vi "_script_fix_vi broken in Tree__JKI_State_Machine_Helper.vi"   [LabVIEW 2014]
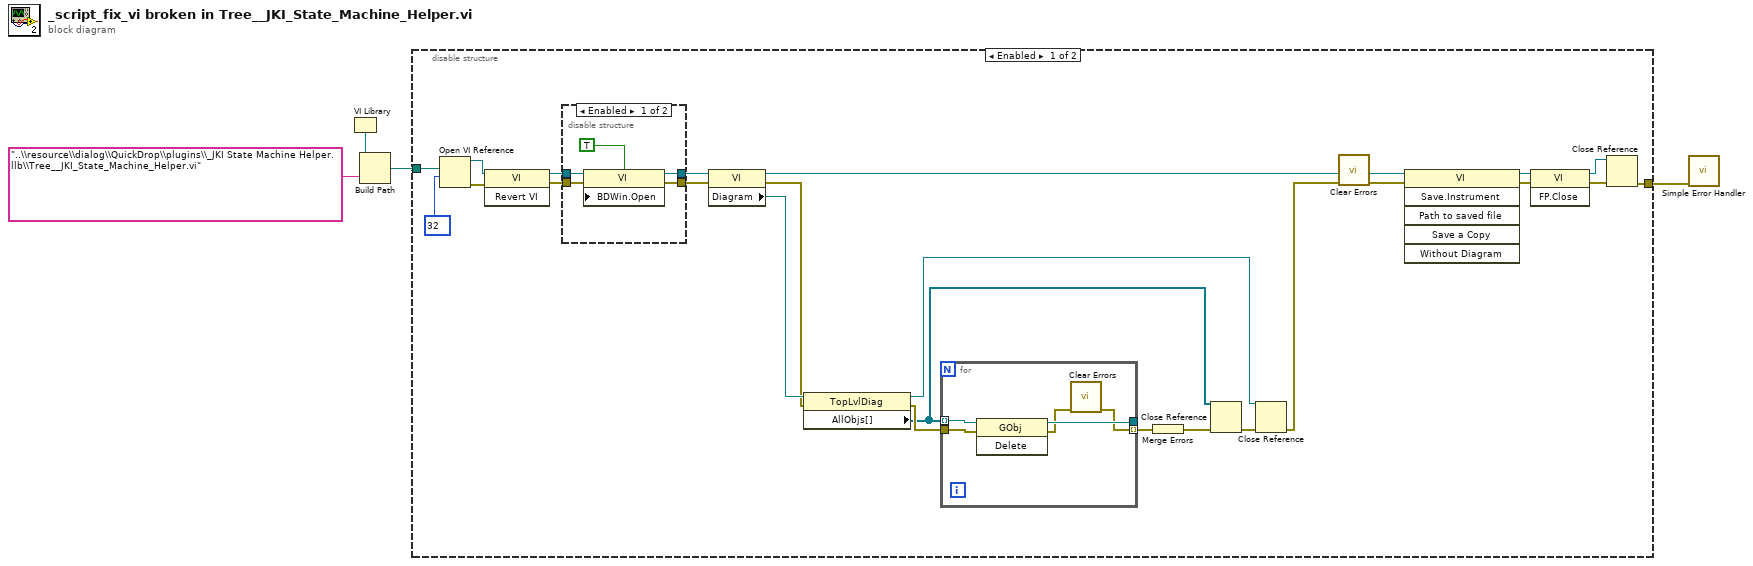
[diagram p0: block diagram]
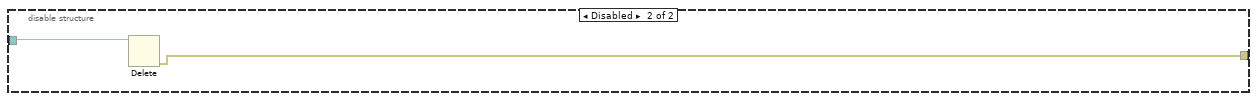
[diagram p3: hidden frame]
diagram:
  n1 = VI Library() -> (path=w4:path)
  n2 = Build Path(base path=w4, name or relative path="..\\resource\\dialog\\QuickDrop\\plugins\\_JKI State Machine Helper.llb\\Tree__JKI_State_Machine_Helper.vi") -> (appended path=w2:path)
  n3 = disable-structure shown="Enabled" {
    disable-tunnel: w2 -> [w26 w42]
    disable-tunnel: [w24 w41] -> w1
    frame Enabled {
      n4 = Open VI Reference(vi path=w26, options=32) -> (vi reference=w27:refnum<vi>, error out=w28:errorcluster)  [unwired: 4 in]
      n5 = invoke class="VI" method="Revert VI"(reference=w27, error in=w28) -> (reference out=w16:refnum<vi>, error out=w15:errorcluster)  [unwired: 1 in, 1 out]
      n6 = disable-structure shown="Enabled" {
        disable-tunnel: w16 -> [w33 w35]
        disable-tunnel: w15 -> [w32 w34]
        disable-tunnel: [w31 w35] -> w14
        disable-tunnel: [w30 w34] -> w13
        frame Enabled {
          n7 = property class="VI"(reference=w33, error in=w32, "BDWin.Open"=TRUE ("Block Diagram Window:Open")) -> (reference out=w31:refnum<vi>, error out=w30:errorcluster)
        }
        frame Disabled {
        }
      }
      n8 = property class="VI"(reference=w14, error in=w13) -> (reference out=w25:refnum<vi>, error out=w22:errorcluster, "Diagram"=w23:refnum<vi>)
      n9 = property class="TopLvlDiag"(reference=w23, error in=w22) -> (reference out=w18:refnum<vi>, error out=w21:errorcluster, "AllObjs[]"=w20:refnum<vi>[])
      n10 = for {
        tunnel: w20 -> [w40] mode=indexing
        tunnel: w21 -> [w39]
        tunnel: [w38] -> _
        tunnel: [w36] -> w7 mode=indexing
        n11 = invoke class="GObj" method="Delete"(reference=w40, error in=w39) -> (reference out=w38:refnum<vi>, error out=w37:errorcluster)  [unwired: 1 in, 1 out]
        n12 = call <vilib>:"Clear Errors.vi"("error in (no error)"=w37) -> ("error out"=w36:errorcluster)  [unwired: 5 in, 1 out]
      }
      n13 = Merge Errors(w7) -> (w6:errorcluster)
      n14 = Close Reference(reference=w20, error in (no error)=w6) -> (error out=w19:errorcluster)
      n15 = Close Reference(reference=w18, error in (no error)=w19) -> (error out=w17:errorcluster)
      n16 = call <vilib>:"Clear Errors.vi"("error in (no error)"=w17) -> ("error out"=w8:errorcluster)  [unwired: 5 in, 1 out]
      n17 = invoke class="VI" method="Save.Instrument"(reference=w25, error in=w8) -> (reference out=w10:refnum<vi>, error out=w12:errorcluster)  [unwired: 4 in, 4 out]
      n18 = invoke class="VI" method="FP.Close"(reference=w10, error in=w12) -> (reference out=w9:refnum<vi>, error out=w11:errorcluster)  [unwired: 1 in, 1 out]
      n19 = Close Reference(reference=w9, error in (no error)=w11) -> (error out=w24:errorcluster)
    }
    frame Disabled {
      n20 = Delete(path (use dialog)=w42) -> (error out=w41:errorcluster)  [unwired: 4 in, 2 out]
    }
  }
  n21 = call <vilib>:"Simple Error Handler.vi"("error in (no error)"=w1) -> ()  [unwired: 4 in, 5 out]
